vi "AWGN(dB)(e5).vi"(10 "AWGN (dB)":dbl, 11 "Dynamic Data":dynamicdata(waveform)) -> (3 "DC with Gaussian Noise":dynamicdata(waveform))   [LabVIEW 2013]
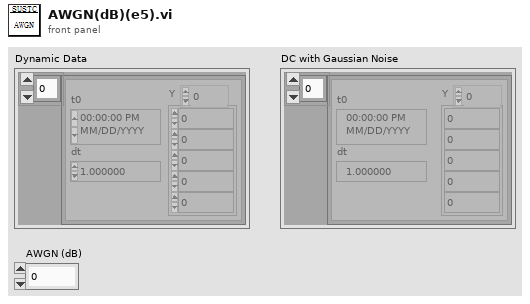
[diagram p1: front panel]
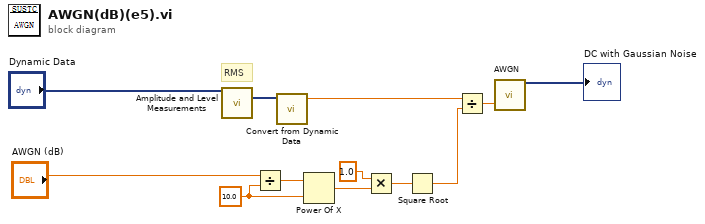
[diagram p0: block diagram]
diagram:
  w3 = 10.0 ("y")
  # "RMS"
  n1 = call "Amplitude and Level Measurements"("Signals"="Dynamic Data") -> ("RMS"=w6:dynamicdata)  [unwired: 13 in, 1 out]
  n2 = Divide(x="AWGN (dB)", y=w3) -> (x/y=w2:dbl)
  n3 = call "Convert from Dynamic Data"("Dynamic Data Type"=w6) -> ("Scalar"=w10:dbl)  [unwired: 3 in]
  n4 = Power Of X(1:w3, 2:w2) -> (0:w11:dbl)
  n5 = Multiply(x=1.0, y=w11) -> (x*y=w7:dbl)
  n6 = Square Root(x=w7) -> (sqrt(x)=w4:dbl)
  n7 = Divide(x=w10, y=w4) -> (x/y=w9:dbl)
  n8 = call "AWGN"("Standard deviation"=w9) -> ("DC with Gaussian Noise"=→"DC with Gaussian Noise":dynamicdata)  [unwired: 13 in, 1 out]
